vi "acknowledgeIRQ.vi"(8 "error in (no error)":errorcluster, 11 "Model in":refnum<class "Model.lvclass">) -> (0 "error out":errorcluster, 3 "Model out":refnum<class "Model.lvclass">)   [LabVIEW 2016, in "Model.lvclass"]
uses:
  Model.lvclass
  Model.lvclass/Model.ctl
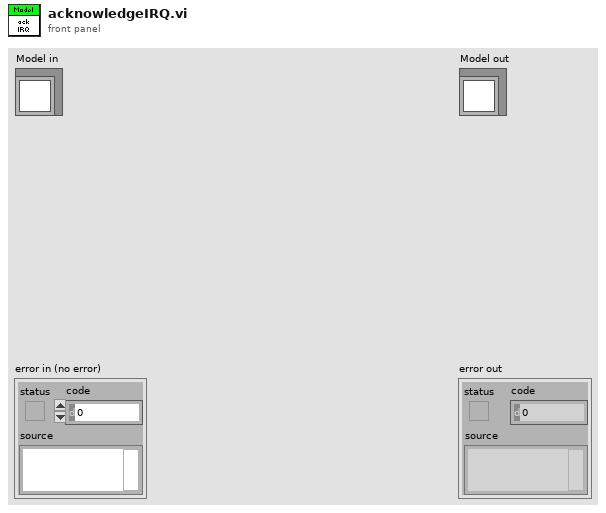
[diagram p1: front panel]
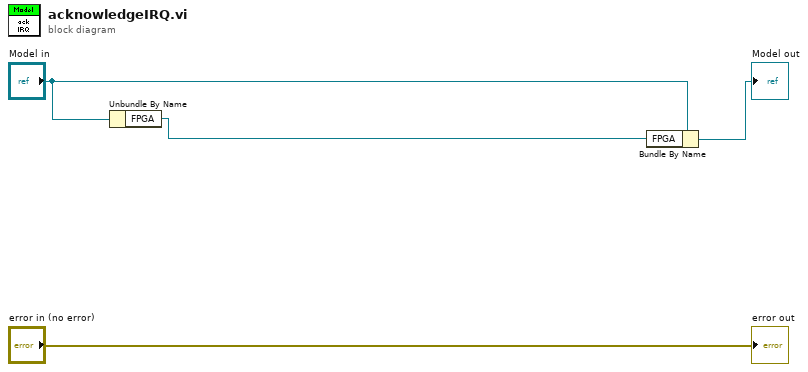
[diagram p0: block diagram]
diagram:
  n1 = Unbundle By Name("Model in") -> ("FPGA"=w4:refnum<class "FPGA.lvclass">)
  n2 = Bundle By Name(cluster="Model in", "FPGA"=w4) -> (→"Model out":refnum<class "Model.lvclass">)
  "error out" <- "error in (no error)"
